vi "Build Path.vi"(8 "error in":errorcluster, 11 "Report Generator in":refnum<class "Report Generator.lvclass">) -> (0 "error out":errorcluster, 3 "Report Generator out":refnum<class "Report Generator.lvclass">)   [LabVIEW 2018, in "Report Generator.lvlib" / "Report Generator.lvclass"]
uses:
  Report Generator.lvclass
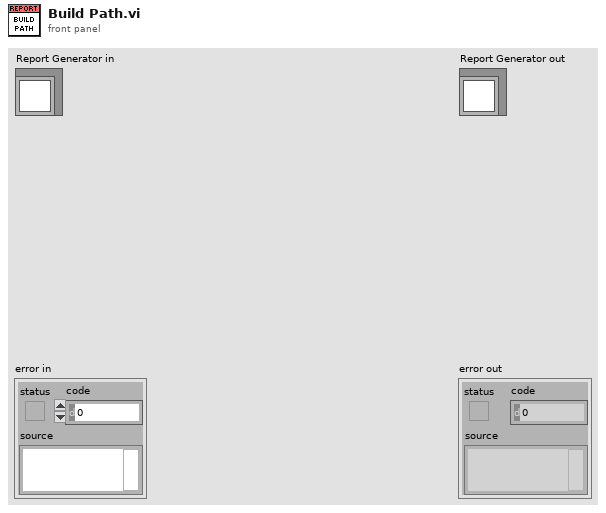
[diagram p1: front panel]
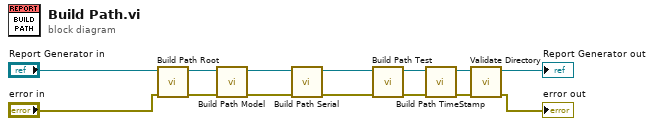
[diagram p0: block diagram]
diagram:
  n1 = call "Build Path Root.vi"("error in"="error in", "Report Generator in"="Report Generator in") -> ("error out"=w9:errorcluster, "Report Generator out"=w13:refnum<class "Report Generator.lvclass">)  [unwired: 8 in]
  n2 = call "Build Path Model.vi"("error in"=w9, "Report Generator in"=w13) -> ("error out"=w8:errorcluster, "Report Generator out"=w12:refnum<class "Report Generator.lvclass">)  [unwired: 8 in]
  n3 = call "Build Path Serial.vi"("error in"=w8, "Report Generator in"=w12) -> ("error out"=w7:errorcluster, "Report Generator out"=w11:refnum<class "Report Generator.lvclass">)  [unwired: 8 in]
  n4 = call "Build Path Test.vi"("error in"=w7, "Report Generator in"=w11) -> ("error out"=w6:errorcluster, "Report Generator out"=w10:refnum<class "Report Generator.lvclass">)  [unwired: 8 in]
  n5 = call "Build Path TimeStamp.vi"("error in"=w6, "Report Generator in"=w10) -> ("error out"=w4:errorcluster, "Report Generator out"=w3:refnum<class "Report Generator.lvclass">)  [unwired: 8 in]
  n6 = call "Validate Directory.vi"("error in (no error)"=w4, "Report Generator in"=w3) -> ("error out"=→"error out":errorcluster, "Report Generator out"=→"Report Generator out":refnum<class "Report Generator.lvclass">)  [unwired: 8 in]
